vi "Corr Digitizer Edit Panel.vi"(6 "current ADC idns":string[](array[string]), 7 "last folder":path caption="Correction file path", 8 "error in":errorcluster, 10 "type":T1 caption="correction type", 11 "path corr":path caption="Correction file path") -> (0 "error out":errorcluster, 3 "path corr out":path caption="Correction file path", 5 "last folder out":path caption="Correction file path")   [LabVIEW 2020]
doc: "Digitizer correction panel. Note: it is recoursive, so it is used for digitizer and channel correction."
uses:
  Corr Digitizer INFO item.ctl
  Corr Digitizer INFO parameter.ctl
  Corr CSV Template.ctl
  Corr Digitizer Parameter Selector.ctl
  Corr Digitizer Type.ctl
  <vilib>/Utility/miscctls.llb/LVRowAndColumnTypeDef.ctl
  Corr Digitizer INFO.ctl
  varilib/varilib.lvlib
panel:
  in  "btn cor info":bool
  in  "btn clear cor":bool
  in  "btn clear par":bool
  in  "disable":bool caption="Disable correction"
  in  "chn name":string caption="Channel name filter (optional)"
  in  "param values":string caption="Parameter values"
  in  "Parameter name":string
  in  "Interpolable parameter":bool
  in  "Parameter":T2
  in  "filter list":i32(listbox) caption="Valid for attribute (right click menu)"
  in  "filter data":string caption="Attribute values (one per row)"
  in  "unc":string[][](table) caption="Uncertainty (right click menu)"
  in  "value":string[][](table) caption="Value (right click menu)"
  out "items":T3[](array[typedef])
  in  "chn list":i32(listbox) caption="Channels list - relative paths to channel corrections (right click menu)"
  in  "chn idns":string caption="Channel identifiers (one channel per row) (right click menu)"
  in  "btn save":bool
  in  "btn ok":bool
  in  "Name":string
  in  "Correction item":u16(ring) items=["interchannel timeshift", "timebase correction"]
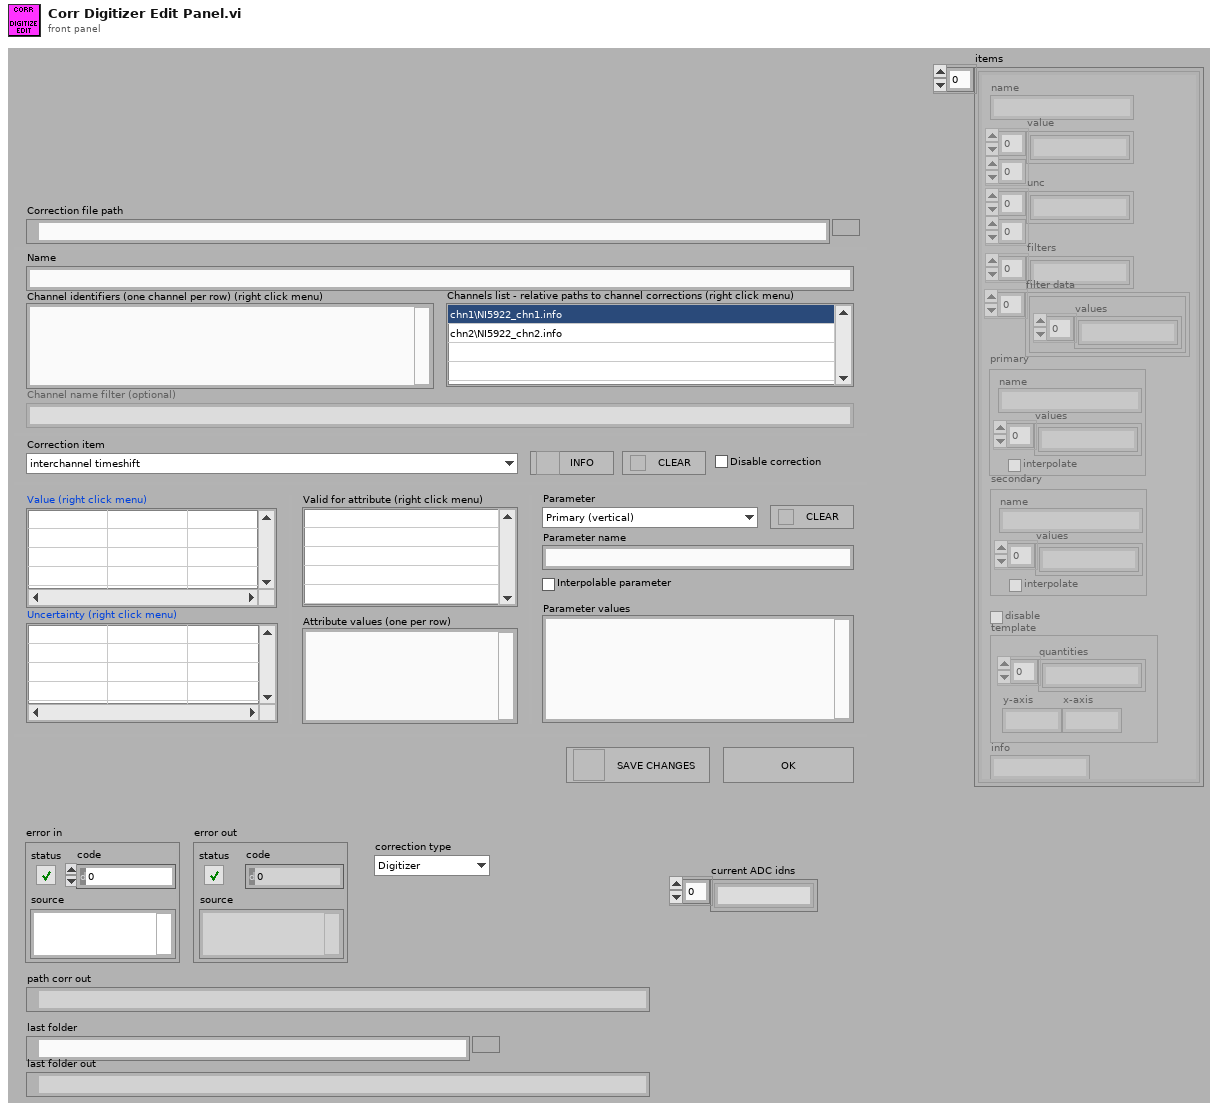
[diagram p1: front panel]
types:
  T1 = typedef "Corr Digitizer Type.ctl" = enum16{"Digitizer", "Channel"}
  T2 = typedef "Corr Digitizer Parameter Selector.ctl" = enum16{"Primary (vertical)", "Secondary (horizontal)"}
  T3 = typedef "Corr Digitizer INFO item.ctl" = cluster{"name":string, "value":string[][], "unc":string[][], "filters":string[], "primary":T4, "secondary":T4, "filter data":cluster{"values":string[]}[], "disable":bool, "template":T5, "info":string}
  T4 = typedef "Corr Digitizer INFO parameter.ctl" = cluster{"values":string[], "interpolate":bool, "name":string}
  T5 = typedef "Corr CSV Template.ctl" = cluster{"quantities":string[], "y-axis":string, "x-axis":string}
  T6 = typedef "Corr Digitizer INFO.ctl" = cluster{"name":string, "identifiers":string[], "channel files":string[], "items":T3[], "channel filter":string}
  T7 = typedef "LVRowAndColumnTypeDef.ctl" = cluster{"Row":i32, "Column":i32}
  T8 = typedef "LVRowAndColumnUnsignedTypeDef.ctl" = cluster{"Row":u32, "Column":u32}
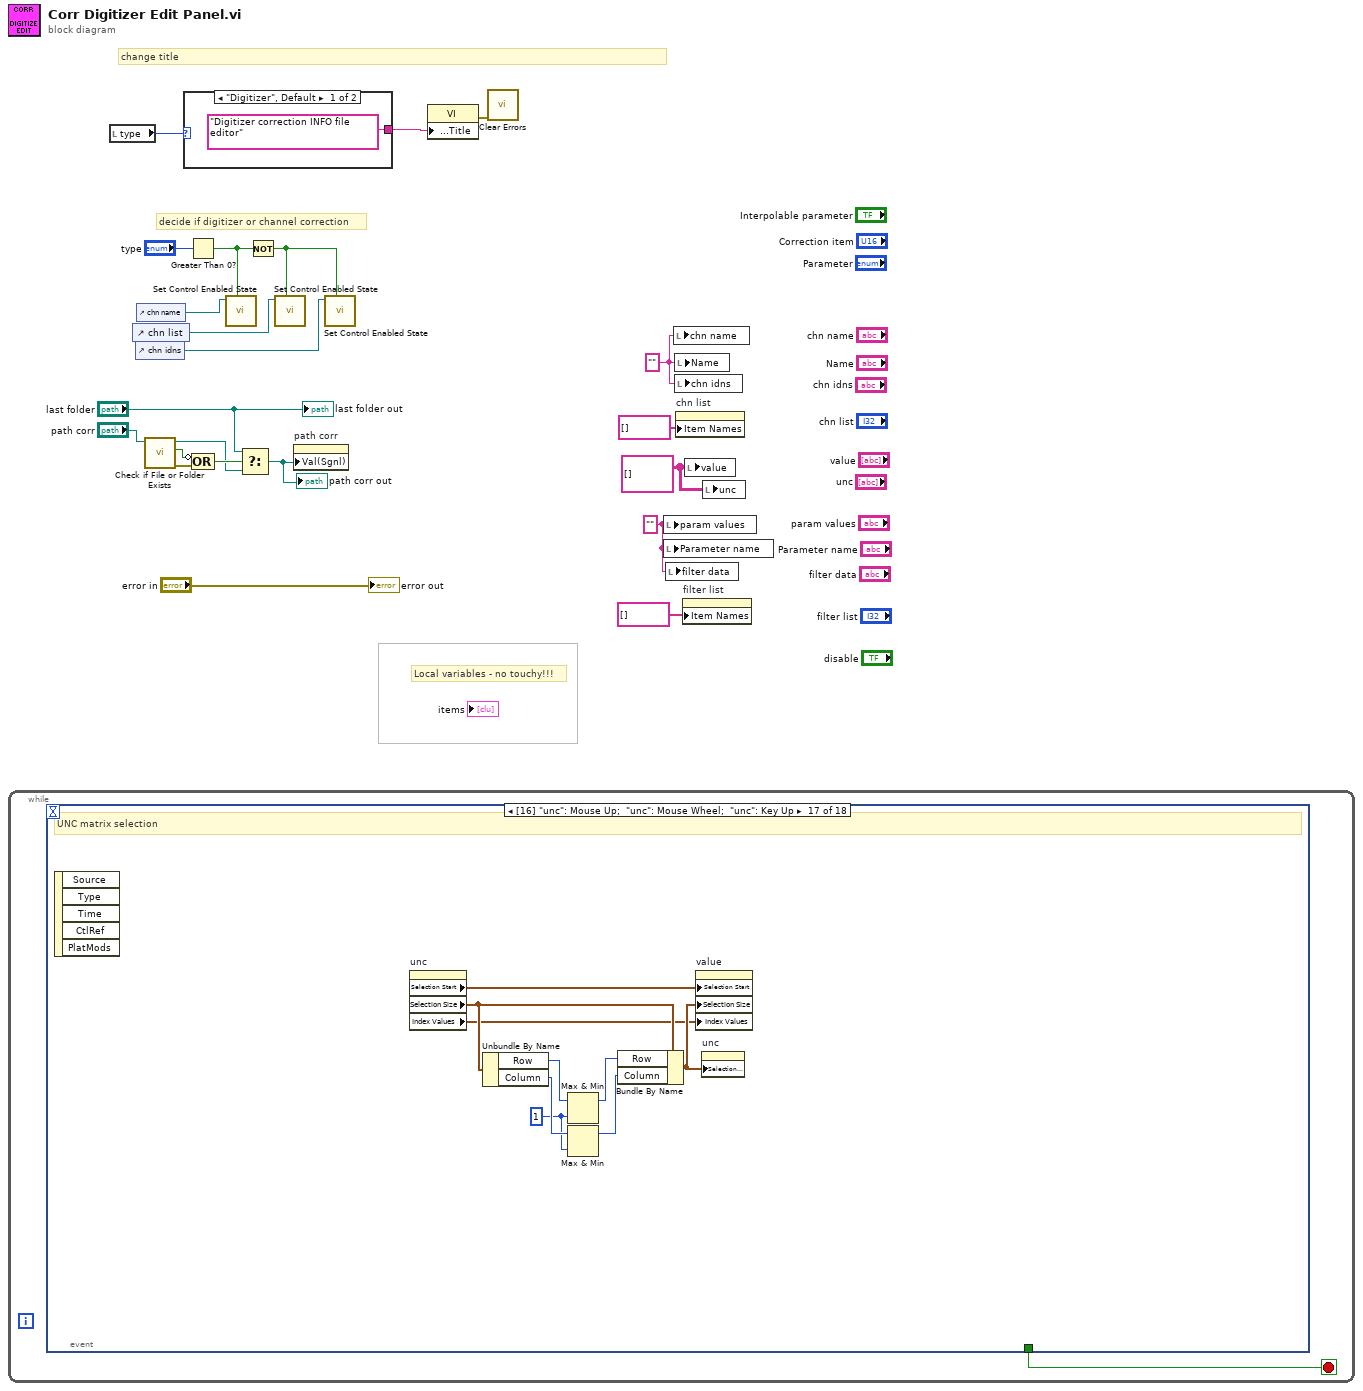
[diagram p0: block diagram]
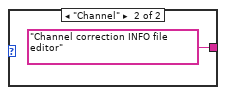
[diagram p2: hidden frame]
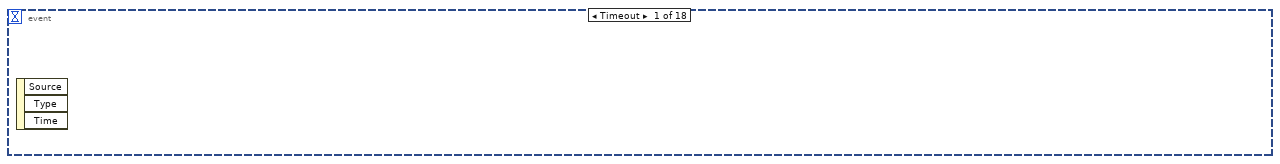
[diagram p3: hidden frame]
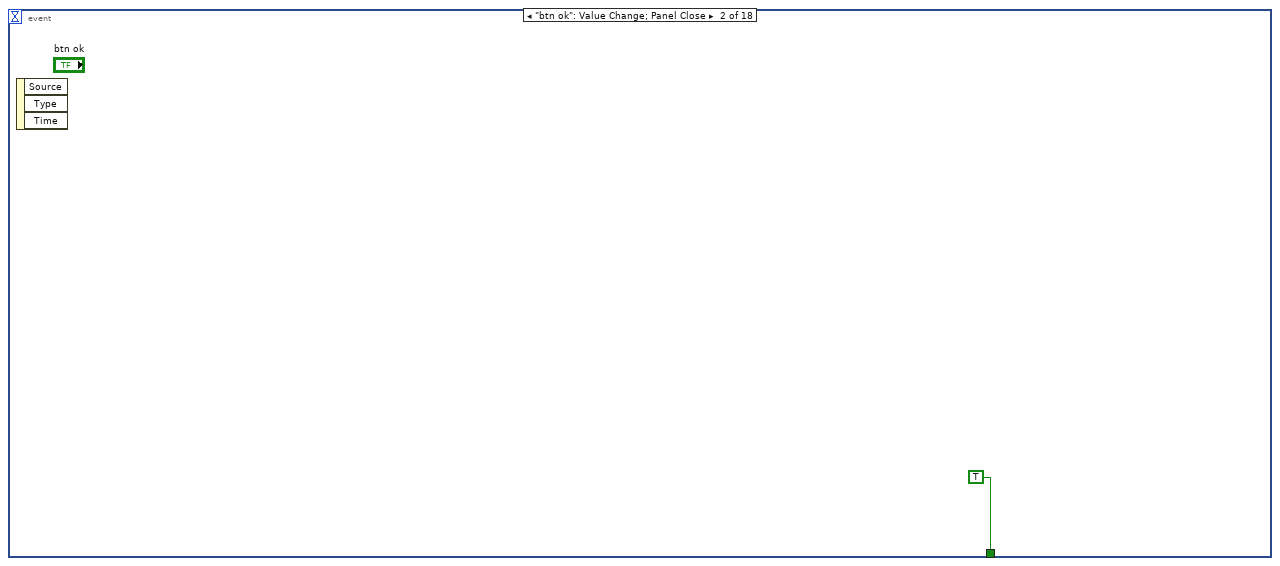
[diagram p4: hidden frame]
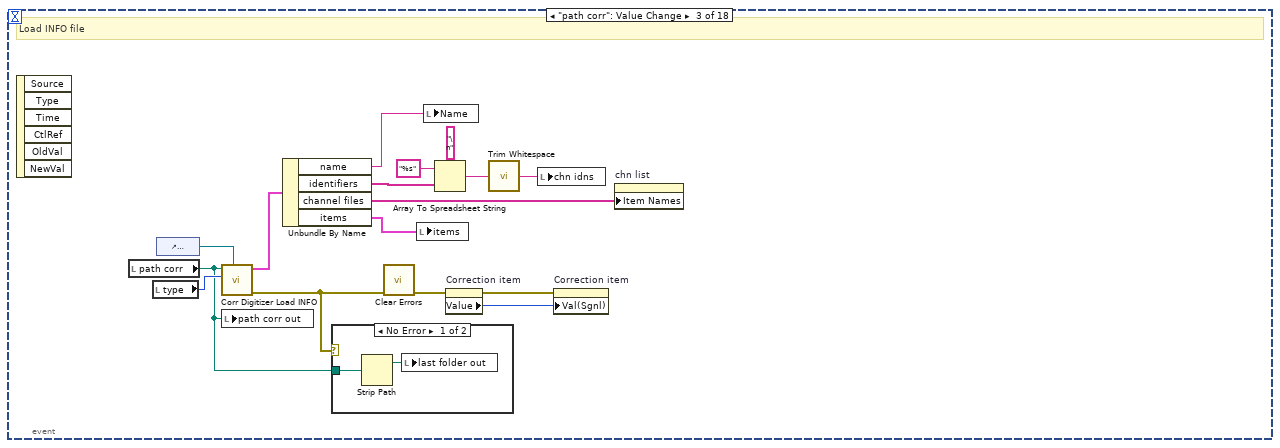
[diagram p5: hidden frame]
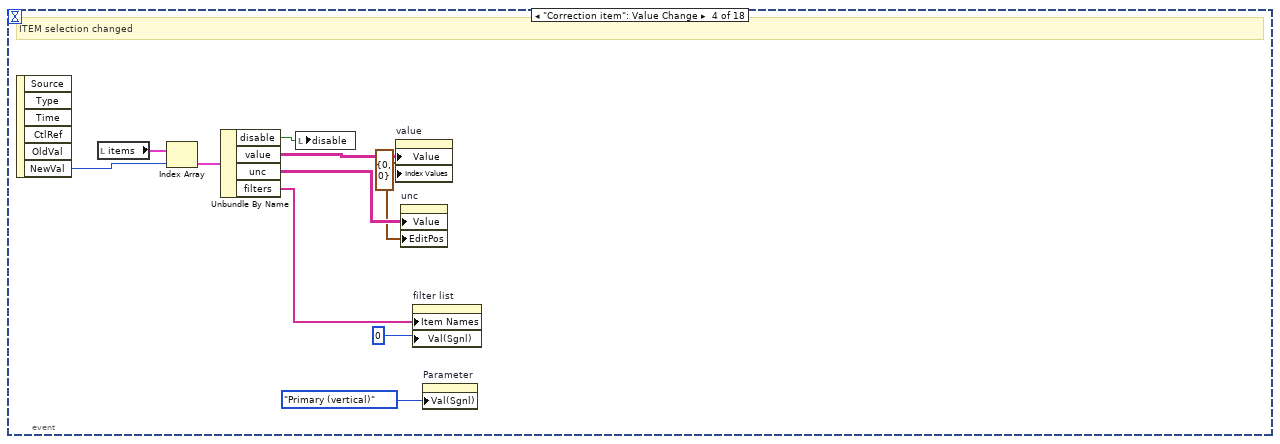
[diagram p7: hidden frame]
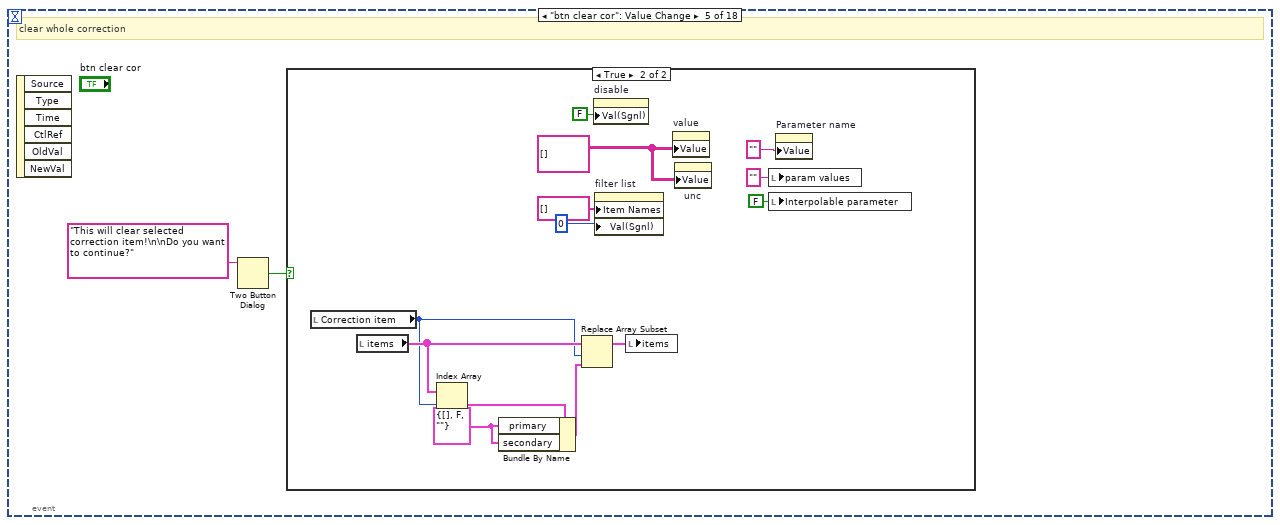
[diagram p8: hidden frame]
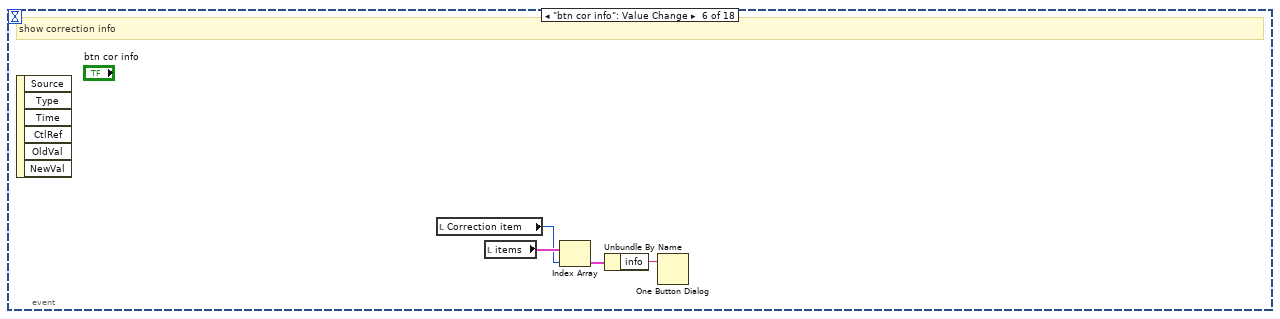
[diagram p10: hidden frame]
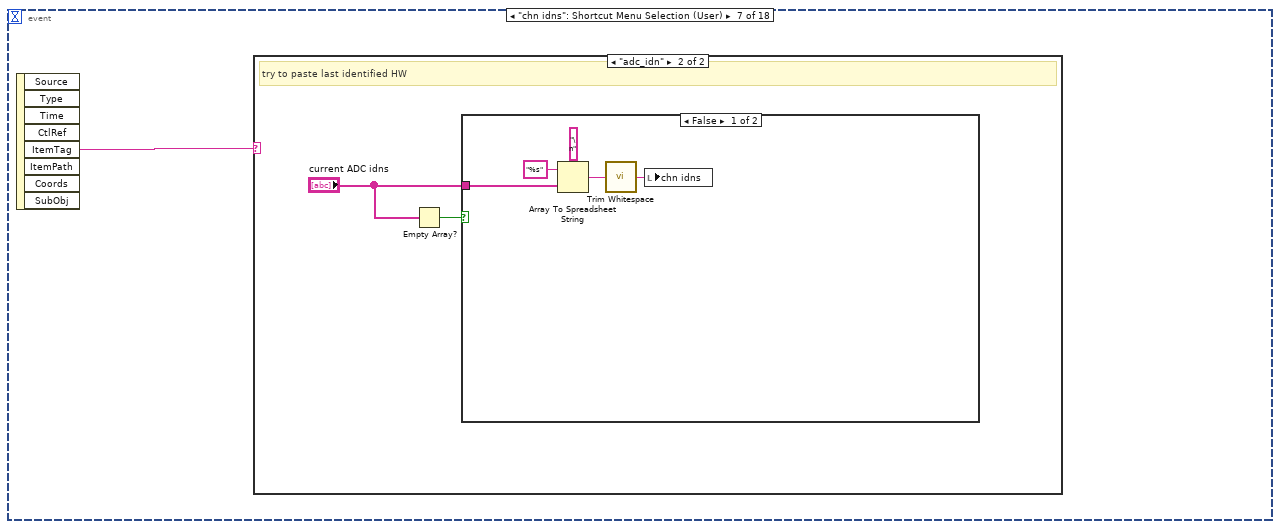
[diagram p11: hidden frame]
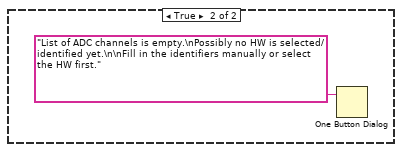
[diagram p13: hidden frame]
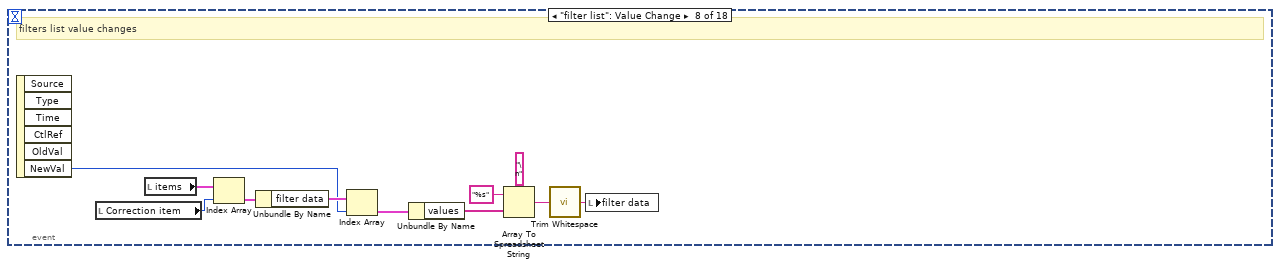
[diagram p14: hidden frame]
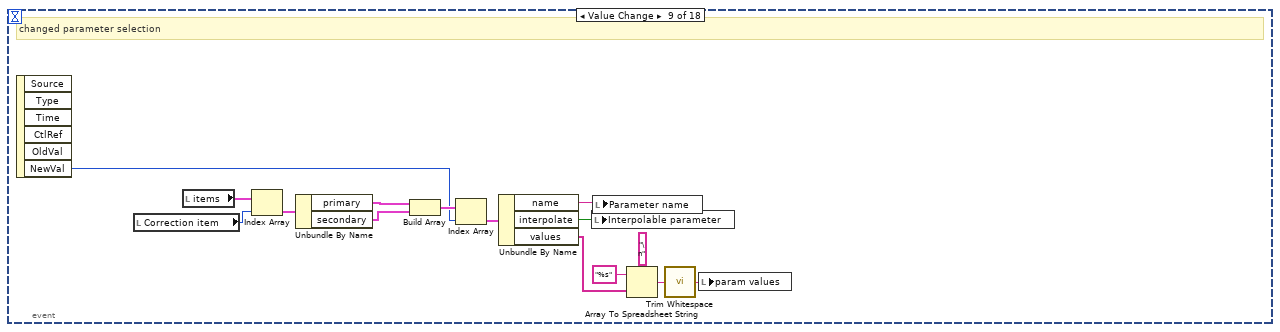
[diagram p15: hidden frame]
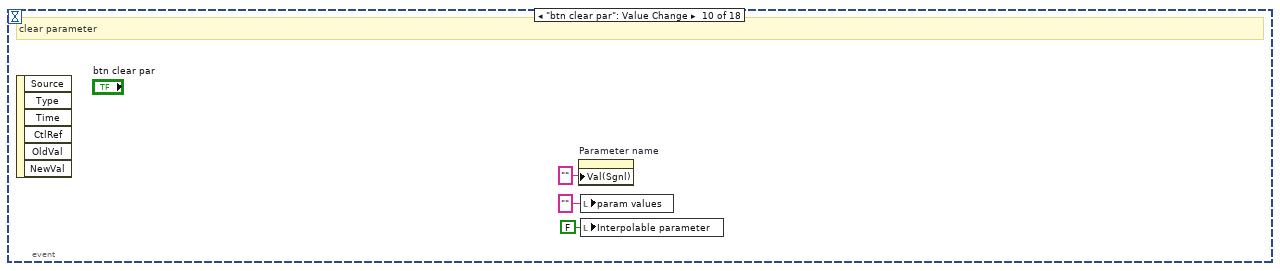
[diagram p16: hidden frame]
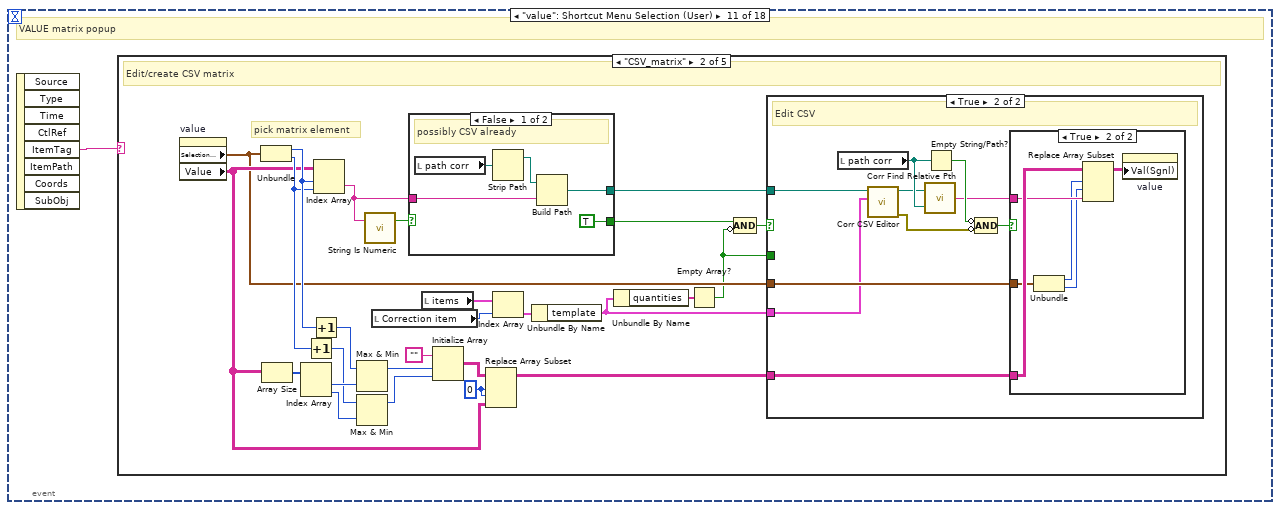
[diagram p17: hidden frame]
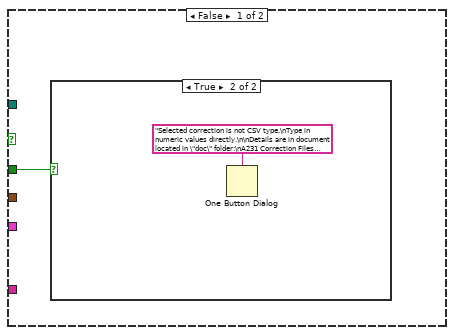
[diagram p19: hidden frame]
diagram:
  w19 = "" ("param values")
  w20 = string[][] [] ("Value")
  w11 = "" ("Type")
  # "change title"
  # "Local variables - no touchy!!!"
  # "decide if digitizer or channel correction"
  n1 = while {
    stop <- w23 stop-if-true
    n2 = event shown="[16] \"unc\": Mouse Up;  \"unc\": Mouse Wheel;  \"unc\": Key Up" {
      selector: _ -> [_ _ _ _ _ _ _ _ _ _ _ _ _ _ _ _ _ _]
      dyn-events: _ -> [_ _ _ _ _ _ _ _ _ _ _ _ _ _ _ _ _ _]
      timeout: _ -> [_ _ _ _ _ _ _ _ _ _ _ _ _ _ _ _ _ _]
      tunnel: [_ TRUE _ _ _ _ _ _ _ _ _ _ _ _ _ _ _ _] -> w23
      event Timeout {
        n3 = event-data() -> ()  [unwired: 1 in, 3 out]
      }
      event "btn ok": Value Change; Panel Close {
        n4 = event-data() -> ()  [unwired: 1 in, 3 out]
      }
      event "path corr": Value Change {
        # "Load INFO file"
        n5 = event-data() -> ()  [unwired: 1 in, 6 out]
        n6 = local read "path corr"() -> (w25:path)
        n7 = local read "type"() -> (w27:T1)
        n8 = control-ref of="Correction item"() -> (w38:refnum<vi>)
        n9 = call "Corr Digitizer Load INFO.vi"("item ref"=w38, "correction type"=w27, "Path"=w25) -> ("error out"=w26:errorcluster, "digitizer info"=w40:T6)  [unwired: 7 in]
        n10 = local write "path corr out"(w25) -> ()
        n11 = Unbundle By Name(w40) -> ("name"=w39:string, "identifiers"=w32:string[], "channel files"=w34:string[], "items"=w33:T3[])
        n12 = case shown="No Error" w26 {
          tunnel: w25 -> [w42 _]
          frame No Error {
            n13 = Strip Path(path=w42) -> (stripped path=w41:path)  [unwired: 1 out]
            n14 = local write "last folder out"(w41) -> ()
          }
          frame Error {
          }
        }
        n15 = call <vilib>:"Clear Errors.vi"("error in (no error)"=w26) -> ("error out"=w37:errorcluster)  [unwired: 5 in, 1 out]
        n16 = local write "items"(w33) -> ()
        n17 = local write "Name"(w39) -> ()
        n18 = Array To Spreadsheet String(delimiter (Tab)="\n", array=w32, 3:"%s" ("format string")) -> (spreadsheet string=w30:string)
        n19 = property on="Correction item" class="Ring (strict)"(error in=w37) -> (error out=w36:errorcluster, "Value"=w35:u16)  [unwired: 1 in, 1 out]
        n20 = call <vilib>:"Trim Whitespace.vi"("string"=w30) -> ("trimmed string"=w28:string)  [unwired: 1 in]
        n21 = local write "chn idns"(w28) -> ()
        n22 = property on="Correction item" class="Ring (strict)"(error in=w36, "Val(Sgnl)"=w35) -> ()  [unwired: 1 in, 2 out]
        n23 = property on="chn list" class="LstBox (strict)"("Item Names"=w34) -> ()  [unwired: 2 in, 2 out]
      }
      event "Correction item": Value Change {
        w43 = T7 {"Row"=0, "Column"=0} ("Edit Position")
        # "ITEM selection changed"
        n24 = event-data() -> ("NewVal"=w52:u16)  [unwired: 1 in, 5 out]
        n25 = local read "items"() -> (w50:T3[])
        n26 = Index Array(array=w50, index=w52) -> (element=w51:T3)
        n27 = Unbundle By Name(w51) -> ("disable"=w46:bool, "value"=w45:string[][], "unc"=w44:string[][], "filters"=w49:string[])
        n28 = local write "disable"(w46) -> ()
        n29 = property on="value" class="Tbl (strict)"("Value"=w45, "Index Values"=w43) -> ()  [unwired: 2 in, 2 out]
        n30 = property on="unc" class="Tbl (strict)"("Value"=w44, "EditPos"=w43) -> ()  [unwired: 2 in, 2 out]
        n31 = property on="filter list" class="LstBox (strict)"("Item Names"=w49, "Val(Sgnl)"=0 ("Value (Signaling)")) -> ()  [unwired: 2 in, 2 out]
        n32 = property on="Parameter" class="Enum (strict)"("Val(Sgnl)"=Corr_Digitizer_Parameter_Selector."Primary (vertical)" ("Value (Signaling)")) -> ()  [unwired: 2 in, 2 out]
      }
      event "btn clear cor": Value Change {
        # "clear whole correction"
        n33 = event-data() -> ()  [unwired: 1 in, 6 out]
        n34 = Two Button Dialog(message="This will clear selected correction item!\n\nDo you want to continue?") -> (T button?=w54:bool)  [unwired: 2 in]
        n35 = case shown="True" w54 {
          frame False {
          }
          frame True {
            w56 = T4 {"values"=[], "interpolate"=FALSE, "name"=""} ("primary")
            w55 = string[][] [] ("value")
            n36 = local read "Correction item"() -> (w59:u16)
            n37 = local read "items"() -> (w60:T3[])
            n38 = Index Array(array=w60, index=w59) -> (element=w58:T3)
            n39 = Bundle By Name(cluster=w58, "primary"=w56, "secondary"=w56) -> (w57:T3)
            n40 = Replace Array Subset(array=w60, new element=w57, index=w59) -> (w64:T3[])
            n41 = property on="disable" class="Bool (strict)"("Val(Sgnl)"=FALSE ("Value (Signaling)")) -> ()  [unwired: 2 in, 2 out]
            n42 = property on="filter list" class="LstBox (strict)"("Item Names"=string[] [], "Val(Sgnl)"=0 ("Value (Signaling)")) -> ()  [unwired: 2 in, 2 out]
            n43 = local write "items"(w64) -> ()
            n44 = property on="value" class="Tbl (strict)"("Value"=w55) -> ()  [unwired: 2 in, 2 out]
            n45 = property on="unc" class="Tbl (strict)"("Value"=w55) -> ()  [unwired: 2 in, 2 out]
            n46 = local write "param values"("" ("param values")) -> ()
            n47 = local write "Interpolable parameter"(FALSE ("disable")) -> ()
            n48 = property on="Parameter name" class="Str"("Value"="" ("Value (Signaling)")) -> ()  [unwired: 2 in, 2 out]
          }
        }
      }
      event "btn cor info": Value Change {
        # "show correction info"
        n49 = event-data() -> ()  [unwired: 1 in, 6 out]
        n50 = local read "Correction item"() -> (w70:u16)
        n51 = local read "items"() -> (w71:T3[])
        n52 = Index Array(array=w71, index=w70) -> (element=w69:T3)
        n53 = Unbundle By Name(w69) -> ("info"=w68:string)
        n54 = One Button Dialog(message=w68) -> ()  [unwired: 1 in, 1 out]
      }
      event "chn idns": Shortcut Menu Selection (User) {
        n55 = event-data() -> ("ItemTag"=w72:string)  [unwired: 1 in, 7 out]
        n56 = case shown="\"adc_idn\"" w72 {
          frame Default {
          }
          frame "adc_idn" {
            # "try to paste last identified HW"
            n57 = Empty Array?(array="current ADC idns") -> (empty?=w74:bool)
            n58 = case shown="False" w74 {
              tunnel: "current ADC idns" -> [w79 _]
              frame False {
                n59 = Array To Spreadsheet String(delimiter (Tab)="\n", array=w79, 3:"%s" ("format string")) -> (spreadsheet string=w76:string)
                n60 = call <vilib>:"Trim Whitespace.vi"("string"=w76) -> ("trimmed string"=w75:string)  [unwired: 1 in]
                n61 = local write "chn idns"(w75) -> ()
              }
              frame True {
                n62 = One Button Dialog(message="List of ADC channels is empty.\nPossibly no HW is selected/identified yet.\n\nFill in the identifiers manually or select the HW first.") -> ()  [unwired: 1 in, 1 out]
              }
            }
          }
        }
      }
      event "filter list": Value Change {
        # "filters list value changes"
        n63 = event-data() -> ("NewVal"=w87:i32)  [unwired: 1 in, 5 out]
        n64 = local read "Correction item"() -> (w89:u16)
        n65 = local read "items"() -> (w90:T3[])
        n66 = Index Array(array=w90, index=w89) -> (element=w91:T3)
        n67 = Unbundle By Name(w91) -> ("filter data"=w88:cluster{"values":string[]}[])
        n68 = Index Array(array=w88, index=w87) -> (element=w86:cluster{"values":string[]})
        n69 = Unbundle By Name(w86) -> ("values"=w82:string[])
        n70 = Array To Spreadsheet String(delimiter (Tab)="\n", array=w82, 3:"%s" ("format string")) -> (spreadsheet string=w84:string)
        n71 = call <vilib>:"Trim Whitespace.vi"("string"=w84) -> ("trimmed string"=w81:string)  [unwired: 1 in]
        n72 = local write "filter data"(w81) -> ()
      }
      event Value Change {
        # "changed parameter selection"
        n73 = event-data() -> ("NewVal"=w99:T2)  [unwired: 1 in, 5 out]
        n74 = local read "Correction item"() -> (w104:u16)
        n75 = local read "items"() -> (w105:T3[])
        n76 = Index Array(array=w105, index=w104) -> (element=w106:T3)
        n77 = Unbundle By Name(w106) -> ("primary"=w102:T4, "secondary"=w101:T4)
        n78 = Build Array(w102, w101) -> (w100:T4[])
        n79 = Index Array(array=w100, index=w99) -> (element=w103:T4)
        n80 = Unbundle By Name(w103) -> ("name"=w98:string, "interpolate"=w97:bool, "values"=w93:string[])
        n81 = local write "Interpolable parameter"(w97) -> ()
        n82 = local write "Parameter name"(w98) -> ()
        n83 = Array To Spreadsheet String(delimiter (Tab)="\n", array=w93, 3:"%s" ("format string")) -> (spreadsheet string=w95:string)
        n84 = call <vilib>:"Trim Whitespace.vi"("string"=w95) -> ("trimmed string"=w92:string)  [unwired: 1 in]
        n85 = local write "param values"(w92) -> ()
      }
      event "btn clear par": Value Change {
        # "clear parameter"
        n86 = event-data() -> ()  [unwired: 1 in, 6 out]
        n87 = property on="Parameter name" class="Str"("Val(Sgnl)"="" ("Value (Signaling)")) -> ()  [unwired: 2 in, 2 out]
        n88 = local write "param values"("" ("param values")) -> ()
        n89 = local write "Interpolable parameter"(FALSE ("disable")) -> ()
      }
      event "value": Shortcut Menu Selection (User) {
        # "VALUE matrix popup"
        n90 = event-data() -> ("ItemTag"=w110:string)  [unwired: 1 in, 7 out]
        n91 = case shown="\"CSV_matrix\"" w110 {
          frame Default {
          }
          frame "CSV_matrix" {
            w120 = 0 ("index (row)")
            # "pick matrix element"
            # "Edit/create CSV matrix"
            n92 = property on="value" class="Tbl (strict)"() -> ("Selection Start"=w119:T7, "Value"=w121:string[][])  [unwired: 2 in, 2 out]
            n93 = Unbundle(w119) -> ("Row"=w132:i32, "Column"=w129:i32)
            n94 = Array Size(array=w121) -> (size(s)=w133:i32[])
            n95 = Index Array(array=w133) -> (element #1=w131:i32, element #2=w130:i32)  [unwired: 2 in]
            n96 = Increment(x=w129) -> (x+1=w127:i32)
            n97 = Increment(x=w132) -> (x+1=w128:i32)
            n98 = Index Array(array=w121, index (row)=w132, index (col)=w129) -> (element=w135:string)
            n99 = Max & Min(x=w128, y=w131) -> (max(x,y)=w125:i32)  [unwired: 1 out]
            n100 = Max & Min(x=w127, y=w130) -> (max(x,y)=w124:i32)  [unwired: 1 out]
            n101 = call "String Is Numeric.vi"("String"=w135) -> ("is numeric"=w136:bool)  [unwired: 1 in, 1 out]
            n102 = local read "Correction item"() -> (w117:u16)
            n103 = case shown="False" w136 {
              tunnel: [TRUE ("T button?") w160] -> w112
              tunnel: w135 -> [w156 _]
              tunnel: [w155 _] -> w134
              frame False {
                # "possibly CSV already"
                n104 = local read "path corr"() -> (w158:path)
                n105 = Strip Path(path=w158) -> (stripped path=w157:path)  [unwired: 1 out]
                n106 = Build Path(base path=w157, name or relative path=w156) -> (appended path=w155:path)
              }
              frame True {
                # "numeric - override?"
                n107 = Two Button Dialog(message="Selected element seems to be numeric!\nOverride by CSV matrix?") -> (T button?=w160:bool)  [unwired: 2 in]
              }
            }
            n108 = local read "items"() -> (w118:T3[])
            n109 = Initialize Array("", w125, w124) -> (w123:string[][])
            n110 = Replace Array Subset(array=w123, new element=w121, index (row)=w120, index (col)=w120) -> (w122:string[][])
            n111 = Index Array(array=w118, index=w117) -> (element=w116:T3)
            n112 = Unbundle By Name(w116) -> ("template"=w115:T5)
            n113 = Unbundle By Name(w115) -> ("quantities"=w114:string[])
            n114 = Empty Array?(array=w114) -> (empty?=w111:bool)
            n115 = Compound Arithmetic op=AND(w112, invert w111) -> (w113:bool)
            n116 = case shown="True" w113 {
              tunnel: w134 -> [_ w148]
              tunnel: w122 -> [_ w141]
              tunnel: w119 -> [_ w140]
              tunnel: w115 -> [_ w139]
              tunnel: w111 -> [w137 _]
              frame False {
                n117 = case shown="True" w137 {
                  frame False {
                  }
                  frame True {
                    n118 = One Button Dialog(message="Selected correction is not CSV type.\nType in numeric values directly.\n\nDetails are in document located in \"doc\" folder:\nA231 Correction Files Reference Manual") -> ()  [unwired: 1 in, 1 out]
                  }
                }
              }
              frame True {
                # "Edit CSV"
                n119 = local read "path corr"() -> (w147:path)
                n120 = call "Corr CSV Editor.vi"("template"=w139, "File path"=w148) -> ("error out"=w145:errorcluster, "path out"=w146:path)  [unwired: 8 in]
                n121 = call "Corr Find Relative Pth.vi"("INFO path"=w147, "CSV path"=w146) -> ("CSV relative path"=w142:string)
                n122 = Empty String/Path?(string/path=w147) -> (empty?=w144:bool)
                n123 = Compound Arithmetic op=AND(invert w144, invert w145) -> (w143:bool)
                n124 = case shown="True" w143 {
                  tunnel: w142 -> [_ w153]
                  tunnel: w141 -> [_ w154]
                  tunnel: w140 -> [_ w152]
                  frame False {
                  }
                  frame True {
                    n125 = Unbundle(w152) -> ("Row"=w151:i32, "Column"=w150:i32)
                    n126 = Replace Array Subset(array=w154, new element=w153, index (row)=w151, index (col)=w150) -> (w149:string[][])
                    n127 = property on="value" class="Tbl (strict)"("Val(Sgnl)"=w149) -> ()  [unwired: 2 in, 2 out]
                  }
                }
              }
            }
          }
          frame "paste" {
            # "Paste matrix override"
            n128 = control-ref of="value"() -> (w163:refnum<vi>)
            n129 = call "Table Paste Clipboard.vi"("signaling change (False)"=TRUE, "table ref"=w163) -> ()  [unwired: 1 out]
          }
          frame "copy" {
            # "copy cells"
            n130 = control-ref of="value"() -> (w164:refnum<vi>)
            n131 = call "Table Copy To Clipboard.vi"("signaling change (False)"=TRUE, "table ref"=w164) -> ()  [unwired: 1 in, 2 out]
          }
          frame "delete" {
            # "copy cells"
            n132 = control-ref of="value"() -> (w168:refnum<vi>)
            n133 = call "Table Copy To Clipboard.vi"("cut (False)"=TRUE, "signaling change (False)"=TRUE, "table ref"=w168) -> ()  [unwired: 2 out]
          }
        }
      }
      event "unc": Shortcut Menu Selection (User) {
        # "UNC matrix popup"
        n134 = event-data() -> ("ItemTag"=w169:string)  [unwired: 1 in, 7 out]
        n135 = case shown="\"remove\"" w169 {
          frame "False", Default {
          }
          frame "paste" {
            # "Paste command override"
            n136 = control-ref of="unc"() -> (w171:refnum<vi>)
            n137 = call "Table Paste Clipboard.vi"("signaling change (False)"=TRUE, "table ref"=w171) -> ()  [unwired: 1 out]
          }
          frame "copy" {
            # "copy command override"
            n138 = control-ref of="unc"() -> (w173:refnum<vi>)
            n139 = call "Table Copy To Clipboard.vi"("signaling change (False)"=TRUE, "table ref"=w173) -> ()  [unwired: 1 in, 2 out]
          }
          frame "remove" {
            # "cut command override"
            n140 = control-ref of="unc"() -> (w176:refnum<vi>)
            n141 = call "Table Copy To Clipboard.vi"("cut (False)"=TRUE, "signaling change (False)"=TRUE, "table ref"=w176) -> ()  [unwired: 2 out]
          }
        }
      }
      event "value", "unc", "filter data", "param values", "disable", "Parameter name", "Interpolable parameter": Value Change; "filter list": Edit Cell {
        # "item changes"
        n142 = event-data() -> ()  [unwired: 1 in, 4 out]
        n143 = local read "param values"() -> (w194:string)
        n144 = local read "filter data"() -> (w225:string)
        n145 = local read "Correction item"() -> (w208:u16)
        n146 = property on="filter list" class="LstBox (strict)"() -> ("Item Names"=w226:string[], "Value"=w213:i32)  [unwired: 2 in, 2 out]
        n147 = call <vilib>:"Trim Whitespace.vi"("string"=w194) -> ("trimmed string"=w199:string)  [unwired: 1 in]
        n148 = call <vilib>:"Trim Whitespace.vi"("string"=w225) -> ("trimmed string"=w206:string)  [unwired: 1 in]
        n149 = local read "items"() -> (w209:T3[])
        n150 = Spreadsheet String To Array(delimiter (Tab)="\n", format string="%s", spreadsheet string=w199, array type (2D Dbl)=string[] []) -> (array=w195:string[])
        n151 = Index Array(array=w209, index=w208) -> (element=w205:T3)
        n152 = Spreadsheet String To Array(delimiter (Tab)="\n", format string="%s", spreadsheet string=w206, array type (2D Dbl)=string[] []) -> (array=w221:string[])
        n153 = call "String Array Replace Local Decimal Separators 1D.vi"("array in"=w195) -> ("array out"=w185:string[])
        n154 = Unbundle By Name(w205) -> ("filter data"=w215:cluster{"values":string[]}[])
        n155 = call "String Array Replace Local Decimal Separators 1D.vi"("array in"=w221) -> ("array out"=w184:string[])
        n156 = local read "Interpolable parameter"() -> (w200:bool)
        n157 = Unbundle By Name(w205) -> ("primary"=w204:T4, "secondary"=w203:T4)
        n158 = local read "Parameter name"() -> (w201:string)
        n159 = Increment(x=w213) -> (x+1=w219:i32)
        n160 = Index Array(array=w215, index=w213) -> (element=w217:cluster{"values":string[]})
        n161 = Bundle By Name(cluster=w217, "values"=w184) -> (w212:cluster{"values":string[]})
        n162 = Array Size(array=w215) -> (size(s)=w220:i32)
        n163 = local read "Parameter"() -> (w191:T2)
        n164 = Max & Min(x=w220, y=w219) -> (max(x,y)=w218:i32)  [unwired: 1 out]
        n165 = Build Array(w204, w203) -> (w193:T4[])
        n166 = Initialize Array(w217, w218) -> (w216:cluster{"values":string[]}[])
        n167 = Index Array(array=w193, index=w191) -> (element=w202:T4)
        n168 = Bundle By Name(cluster=w202, "name"=w201, "interpolate"=w200, "values"=w185) -> (w192:T4)
        n169 = Replace Array Subset(array=w216, new element=w215) -> (w214:cluster{"values":string[]}[])  [unwired: 1 in]
        n170 = Replace Array Subset(array=w214, new element=w212, index=w213) -> (w211:cluster{"values":string[]}[])
        n171 = Replace Array Subset(array=w193, new element=w192, index=w191) -> (w190:T4[])
        n172 = control-ref of="value"() -> (w182:refnum<vi>)
        n173 = control-ref of="unc"() -> (w178:refnum<vi>)
        n174 = Index Array(array=w190) -> (element #1=w189:T4, element #2=w188:T4)  [unwired: 2 in]
        n175 = call "Table Trim Whites.vi"("table ref"=w182) -> ("error out"=w180:errorcluster, "reduced array"=w181:string[][])  [unwired: 8 in, 1 out]
        n176 = call "Table Trim Whites.vi"("table ref"=w178) -> ("error out"=w179:errorcluster, "reduced array"=w177:string[][])  [unwired: 8 in, 1 out]
        n177 = call <vilib>:"Clear Errors.vi"("error in (no error)"=w180) -> ()  [unwired: 5 in, 2 out]
        n178 = call <vilib>:"Clear Errors.vi"("error in (no error)"=w179) -> ()  [unwired: 5 in, 2 out]
        n179 = local read "disable"() -> (w183:bool)
        n180 = call "String Array Replace Local Decimal Separators 2D.vi"("array in"=w181) -> ("array out"=w187:string[][])
        n181 = call "String Array Replace Local Decimal Separators 2D.vi"("array in"=w177) -> ("array out"=w186:string[][])
        n182 = Bundle By Name(cluster=w205, "value"=w187, "unc"=w186, "filters"=w226, "filter data"=w211, "primary"=w189, "secondary"=w188, "disable"=w183) -> (w210:T3)
        n183 = Replace Array Subset(array=w209, new element=w210, index=w208) -> (w207:T3[])
        n184 = local write "items"(w207) -> ()
      }
      event "filter list": Shortcut Menu Selection (User) {
        # "filter list pupup"
        n185 = event-data() -> ("ItemTag"=w227:string)  [unwired: 1 in, 7 out]
        n186 = case shown="\"clear\"" w227 {
          frame Default {
          }
          frame "remove" {
            w235 = 1 ("length")
            n187 = local read "Correction item"() -> (w231:u16)
            n188 = local read "items"() -> (w233:T3[])
            n189 = Index Array(array=w233, index=w231) -> (element=w238:T3)
            n190 = Unbundle By Name(w238) -> ("filters"=w239:string[], "filter data"=w237:cluster{"values":string[]}[])
            n191 = property on="filter list" class="LstBox (strict)"() -> ("Value"=w234:i32)  [unwired: 2 in, 2 out]
            n192 = Delete From Array(array=w237, length=w235, index=w234) -> (array with subset deleted=w236:cluster{"values":string[]}[])  [unwired: 1 out]
            n193 = Delete From Array(array=w239, length=w235, index=w234) -> (array with subset deleted=w229:string[])  [unwired: 1 out]
            n194 = Bundle By Name(cluster=w238, "filters"=w229, "filter data"=w236) -> (w232:T3)
            n195 = property on="filter list" class="LstBox (strict)"("Item Names"=w229, "Val(Sgnl)"=0 ("Value (Signaling)")) -> ()  [unwired: 2 in, 2 out]
            n196 = Replace Array Subset(array=w233, new element=w232, index=w231) -> (w230:T3[])
            n197 = local write "items"(w230) -> ()
          }
          frame "clear" {
            w241 = string[] [] ("filters")
            n198 = local read "Correction item"() -> (w244:u16)
            n199 = local read "items"() -> (w246:T3[])
            n200 = Index Array(array=w246, index=w244) -> (element=w247:T3)
            n201 = Bundle By Name(cluster=w247, "filters"=w241, "filter data"=cluster{"values":string[]}[] []) -> (w245:T3)
            n202 = property on="filter list" class="LstBox (strict)"("Item Names"=w241, "Val(Sgnl)"=0 ("Value (Signaling)")) -> ()  [unwired: 2 in, 2 out]
            n203 = Replace Array Subset(array=w246, new element=w245, index=w244) -> (w243:T3[])
            n204 = local write "items"(w243) -> ()
          }
          frame "new" {
            n205 = local read "Correction item"() -> (w253:u16)
            n206 = local read "items"() -> (w256:T3[])
            n207 = Index Array(array=w256, index=w253) -> (element=w257:T3)
            n208 = Unbundle By Name(w257) -> ("filter data"=w251:cluster{"values":string[]}[])
            n209 = property on="filter list" class="LstBox (strict)"() -> ("Item Names"=w261:string[])  [unwired: 2 in, 2 out]
            n210 = Bundle(string[] []) -> (w248:cluster{string[]})  [unwired: 1 in]
            n211 = Build Array (concatenate)(w251, w248) -> (w250:cluster{"values":string[]}[])
            n212 = Build Array (concatenate)(w261, ">>> click to edit <<<") -> (w252:string[])
            n213 = Array Size(array=w252) -> (size(s)=w259:i32)
            n214 = Bundle By Name(cluster=w257, "filters"=w252, "filter data"=w250) -> (w255:T3)
            n215 = Decrement(x=w259) -> (x-1=w258:i32)
            n216 = property on="filter list" class="LstBox (strict)"("Item Names"=w252, "Val(Sgnl)"=w258) -> ()  [unwired: 2 in, 2 out]
            n217 = Replace Array Subset(array=w256, new element=w255, index=w253) -> (w254:T3[])
            n218 = local write "items"(w254) -> ()
          }
        }
      }
      event "chn list": Shortcut Menu Selection (User) {
        # "channel list pupup"
        n219 = event-data() -> ("ItemTag"=w262:string)  [unwired: 1 in, 7 out]
        n220 = case shown="\"edit\"" w262 {
          frame Default {
          }
          frame "remove" {
            n221 = property on="chn list" class="LstBox (strict)"() -> ("Value"=w266:i32, "Item Names"=w264:string[])  [unwired: 2 in, 2 out]
            n222 = Delete From Array(array=w264, length=1, index=w266) -> (array with subset deleted=w263:string[])  [unwired: 1 out]
            n223 = property on="chn list" class="LstBox (strict)"("Item Names"=w263, "Val(Sgnl)"=0 ("Value (Signaling)")) -> ()  [unwired: 2 in, 2 out]
          }
          frame "new" {
            n224 = property on="chn list" class="LstBox (strict)"() -> ("Item Names"=w272:string[])  [unwired: 2 in, 2 out]
            n225 = Build Array (concatenate)(w272, ">>> click to edit <<<") -> (w268:string[])
            n226 = Array Size(array=w268) -> (size(s)=w270:i32)
            n227 = Decrement(x=w270) -> (x-1=w269:i32)
            n228 = property on="chn list" class="LstBox (strict)"("Item Names"=w268, "Val(Sgnl)"=w269) -> ()  [unwired: 2 in, 2 out]
          }
          frame "edit" {
            # "recoursive launch of the editor\nfor channel correction"
            # "tryto build channel path"
            n229 = local read "path corr"() -> (w282:path)
            n230 = property on="chn list" class="LstBox (strict)"() -> ("Item Names"=w280:string[], "Value"=w279:i32)  [unwired: 2 in, 2 out]
            n231 = Strip Path(path=w282) -> (stripped path=w281:path)  [unwired: 1 out]
            n232 = Index Array(array=w280, index=w279) -> (element=w278:string)
            n233 = Build Path(base path=w281, name or relative path=w278) -> (appended path=w277:path)
            n234 = call "Corr Digitizer Edit Panel.vi"("type"=Corr_Digitizer_Type."Channel", "path corr"=w277) -> ("error out"=w276:errorcluster, "path corr out"=w273:path)  [unwired: 7 in, 1 out]
            n235 = Empty String/Path?(string/path=w273) -> (empty?=w275:bool)
            n236 = Compound Arithmetic op=AND(invert w276, invert w275) -> (w274:bool)
            n237 = case shown="True" w274 {
              tunnel: w273 -> [_ w292]
              frame False {
              }
              frame True {
                # "success - store channel path to list"
                n238 = local read "path corr"() -> (w291:path)
                n239 = property on="chn list" class="LstBox (strict)"() -> (error out=w285:errorcluster, "Item Names"=w290:string[], "Value"=w288:i32)  [unwired: 2 in, 1 out]
                n240 = call "Corr Find Relative Pth.vi"("INFO path"=w291, "CSV path"=w292) -> ("CSV relative path"=w289:string)
                n241 = Replace Array Subset(array=w290, new element=w289, index=w288) -> (w287:string[])
                n242 = property on="chn list" class="LstBox (strict)"(error in=w285, "Item Names"=w287) -> (error out=w284:errorcluster)  [unwired: 1 in, 1 out]
                n243 = property class="VI"(error in=w284, "Front Panel.Title"="Digitizer correction INFO file editor") -> ()  [unwired: 1 in, 2 out]
              }
            }
          }
        }
      }
      event "value": Mouse Up; "value": Mouse Wheel; "value": Key Up {
        w298 = 1 ("y")
        # "VALUE matrix selection"
        n244 = event-data() -> ()  [unwired: 1 in, 5 out]
        n245 = property on="value" class="Tbl (strict)"() -> ("Selection Start"=w301:T7, "Selection Size"=w295:T7, "Index Values"=w293:T8)  [unwired: 2 in, 2 out]
        n246 = Unbundle By Name(w295) -> ("Row"=w300:i32, "Column"=w299:i32)
        n247 = Max & Min(x=w300, y=w298) -> (max(x,y)=w297:i32)  [unwired: 1 out]
        n248 = Max & Min(x=w299, y=w298) -> (max(x,y)=w296:i32)  [unwired: 1 out]
        n249 = Bundle By Name(cluster=w295, "Row"=w297, "Column"=w296) -> (w294:T7)
        n250 = property on="unc" class="Tbl (strict)"("Selection Start"=w301, "Selection Size"=w294, "Index Values"=w293) -> ()  [unwired: 2 in, 2 out]
        n251 = property on="value" class="Tbl (strict)"("Selection Size"=w294) -> ()  [unwired: 2 in, 2 out]
      }
      event "unc": Mouse Up; "unc": Mouse Wheel; "unc": Key Up {
        w307 = 1 ("y")
        # "UNC matrix selection"
        n252 = event-data() -> ()  [unwired: 1 in, 5 out]
        n253 = property on="unc" class="Tbl (strict)"() -> ("Selection Start"=w310:T7, "Selection Size"=w306:T7, "Index Values"=w302:T8)  [unwired: 2 in, 2 out]
        n254 = Unbundle By Name(w306) -> ("Row"=w309:i32, "Column"=w308:i32)
        n255 = Max & Min(x=w309, y=w307) -> (max(x,y)=w305:i32)  [unwired: 1 out]
        n256 = Max & Min(x=w308, y=w307) -> (max(x,y)=w304:i32)  [unwired: 1 out]
        n257 = Bundle By Name(cluster=w306, "Row"=w305, "Column"=w304) -> (w303:T7)
        n258 = property on="value" class="Tbl (strict)"("Selection Start"=w310, "Selection Size"=w303, "Index Values"=w302) -> ()  [unwired: 2 in, 2 out]
        n259 = property on="unc" class="Tbl (strict)"("Selection Size"=w303) -> ()  [unwired: 2 in, 2 out]
      }
      event "btn save": Value Change {
        # "Save changes"
        n260 = event-data() -> ()  [unwired: 1 in, 6 out]
        n261 = local read "path corr"() -> (w319:path)
        n262 = Strip Path(path=w319) -> (stripped path=w318:path)  [unwired: 1 out]
        n263 = call "File Dialog"("start path"=w318, "prompt"="Select correction file name", "pattern (all files)"="*.info", "pattern label"="Correction INFO file") -> ("selected path"=w311:path, "cancelled"=w313:bool, "error out"=w314:errorcluster)  [unwired: 8 in, 1 out]
        n264 = Compound Arithmetic op=AND(invert w313, invert w314) -> (w312:bool)
        n265 = case shown="True" w312 {
          tunnel: w311 -> [_ w321]
          frame False {
          }
          frame True {
            n266 = property on="chn list" class="LstBox (strict)"() -> ("Item Names"=w328:string[])  [unwired: 2 in, 2 out]
            n267 = local read "chn idns"() -> (w329:string)
            n268 = local read "items"() -> (w331:T3[])
            n269 = local read "chn name"() -> (w323:string)
            n270 = Spreadsheet String To Array(delimiter (Tab)="\n", format string="%s", spreadsheet string=w329, array type (2D Dbl)=string[] []) -> (array=w327:string[])
            n271 = local read "Name"() -> (w330:string)
            n272 = Bundle By Name(cluster=T6 {"name"="", "identifiers"=[], "channel files"=[], "items"=[], "channel filter"=""} ("transducer info"), "name"=w330, "identifiers"=w327, "channel files"=w328, "channel filter"=w323, "items"=w331) -> (w332:T6)
            n273 = local read "path corr"() -> (w322:path)
            n274 = local read "type"() -> (w334:T1)
            n275 = call "Corr Digitizer Save INFO raw.vi"("path template"=w322, "digitizer info"=w332, "correction type"=w334, "path result"=w321) -> ("error out"=w320:errorcluster)  [unwired: 7 in]
            n276 = flat-sequence {
              tunnel: w321 -> [w335]
              tunnel: w320 -> [w337]
              frame #0 {
                n277 = call <vilib>:"Simple Error Handler.vi"("error in (no error)"=w337) -> ("error out"=w336:errorcluster)  [unwired: 4 in, 4 out]
                n278 = case shown="No Error" w336 {
                  tunnel: w335 -> [w338 _]
                  frame No Error {
                    n279 = Strip Path(path=w338) -> (stripped path=w339:path)  [unwired: 1 out]
                    n280 = local write "last folder out"(w339) -> ()
                  }
                  frame Error {
                  }
                }
                n281 = local write "path corr out"(w335) -> ()
                n282 = local write "path corr"(w335) -> ()
              }
            }
          }
        }
      }
    }
  }
  n283 = local read "type"() -> (w3:T1)
  n284 = control-ref of="chn list"() -> (w14:refnum<vi>)
  n285 = control-ref of="chn idns"() -> (w13:refnum<vi>)
  n286 = control-ref of="chn name"() -> (w12:refnum<vi>)
  n287 = call <vilib>:"Check if File or Folder Exists.vi"("path"="path corr") -> ("error out"=w8:errorcluster, "file or folder exists?"=w9:bool, "dup path"=w6:path)  [unwired: 8 in]
  n288 = case shown="\"Digitizer\", Default" w3 {
    tunnel: ["Digitizer correction INFO file editor" "Channel correction INFO file editor"] -> w2
    frame "Digitizer", Default {
    }
    frame "Channel" {
    }
  }
  n289 = Greater Than 0?(x="type") -> (x > 0?=w16:bool)
  n290 = Compound Arithmetic op=OR(invert w9, w8) -> (w7:bool)
  n291 = call "Set Control Enabled State.vi"("enabled (T)"=w16, "reference in"=w12) -> ()  [unwired: 8 in, 2 out]
  n292 = Select(t="last folder", s=w7, f=w6) -> (s? t:f=w5:path)
  "path corr out" <- w5
  n293 = Not(x=w16) -> (.not. x?=w15:bool)
  n294 = call "Set Control Enabled State.vi"("enabled (T)"=w15, "reference in"=w14) -> ()  [unwired: 8 in, 2 out]
  n295 = property on="path corr" class="Path"("Val(Sgnl)"=w5) -> ()  [unwired: 2 in, 2 out]
  n296 = call "Set Control Enabled State.vi"("enabled (T)"=w15, "reference in"=w13) -> ()  [unwired: 8 in, 2 out]
  n297 = property class="VI"("Front Panel.Title"=w2) -> (error out=w1:errorcluster)  [unwired: 2 in, 1 out]
  n298 = call <vilib>:"Clear Errors.vi"("error in (no error)"=w1) -> ()  [unwired: 5 in, 2 out]
  n299 = local write "param values"(w19) -> ()
  n300 = local write "Parameter name"(w19) -> ()
  n301 = local write "filter data"(w19) -> ()
  n302 = local write "chn name"(w11) -> ()
  n303 = local write "Name"(w11) -> ()
  n304 = local write "chn idns"(w11) -> ()
  n305 = property on="chn list" class="LstBox (strict)"("Item Names"=string[] []) -> ()  [unwired: 2 in, 2 out]
  n306 = property on="filter list" class="LstBox (strict)"("Item Names"=string[] []) -> ()  [unwired: 2 in, 2 out]
  n307 = local write "value"(w20) -> ()
  n308 = local write "unc"(w20) -> ()
  "error out" <- "error in"
  "last folder out" <- "last folder"
